vi "To Waveform.vi"(8 "error in (no error)":errorcluster, 11 "U32 Array in":refnum<class "U32 Array.lvclass">) -> (0 "error out":errorcluster, 1 "Success?":bool, 3 "Waveform Array":waveform(dbl)[](array[waveform]))   [LabVIEW 2020, in "Data.lvlib" / "U32 Array.lvclass"]
doc: "Interpret 'Data' as a Waveform Array. If impossible 'Success?' is set to FALSE"
uses:
  U32 Array.lvclass
  U32 Array.lvclass/U32 Array.ctl
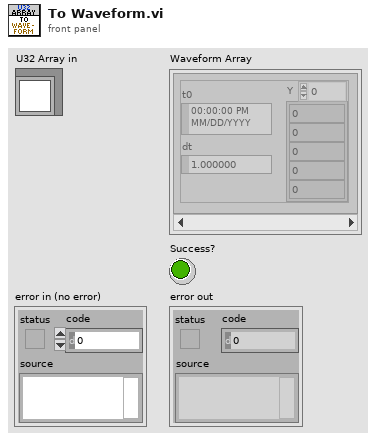
[diagram p1: front panel]
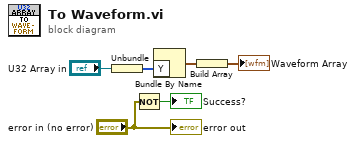
[diagram p0: block diagram]
diagram:
  n1 = Unbundle("U32 Array in") -> (w5:u32[])
  n2 = Not(x="error in (no error)") -> (.not. x?=→"Success?":bool)
  n3 = Bundle By Name("Y"=w5) -> (w6:waveform(u32))  [unwired: 1 in]
  n4 = Build Array(w6) -> (→"Waveform Array":waveform(u32)[])
  "error out" <- "error in (no error)"
